vi "Rotation3d_GetXYZ.vi"(11 "in Rotation3d":T1={"Q_quaternion"={"R"=1.0, "V"=[0.0, 0.0, 0.0]}}) -> (1 "Z":dbl, 2 "Y":dbl, 3 "X":dbl)   [LabVIEW 2019, in "Trajectory_Library.lvlib"]
doc: "Returns the counterclockwise rotation angle around the X axis (roll) in radians and the counterclockwise rotation angle around the Y axis (pitch) in radians and the counterclockwise rotation angle around the Z axis (yaw) in radians.\n\nParameters:\n - in ROTATION3D - This ROTATION3D data structure\n\nReturns:\n - X -- The counterclockwise rotation angle around the X axis (roll) in radians.\n - Y -- The counterclockwise rotation angle around the Y axis (pitch) in radians.\n - Z -- The counterclockwise rotation angle around the Z axis (yaw) in radians."
uses:
  Trajectory_Library.lvlib
  TypeDef/ROTATION3D.ctl
  TypeDef/QUATERNION.ctl
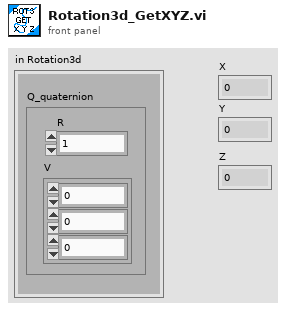
[diagram p1: front panel]
types:
  T1 = typedef "Trajectory_Library.lvlib/ROTATION3D.ctl" = cluster{"Q_quaternion":T2}
  T2 = typedef "Trajectory_Library.lvlib/QUATERNION.ctl" = cluster{"R":dbl, "V":dbl[]}
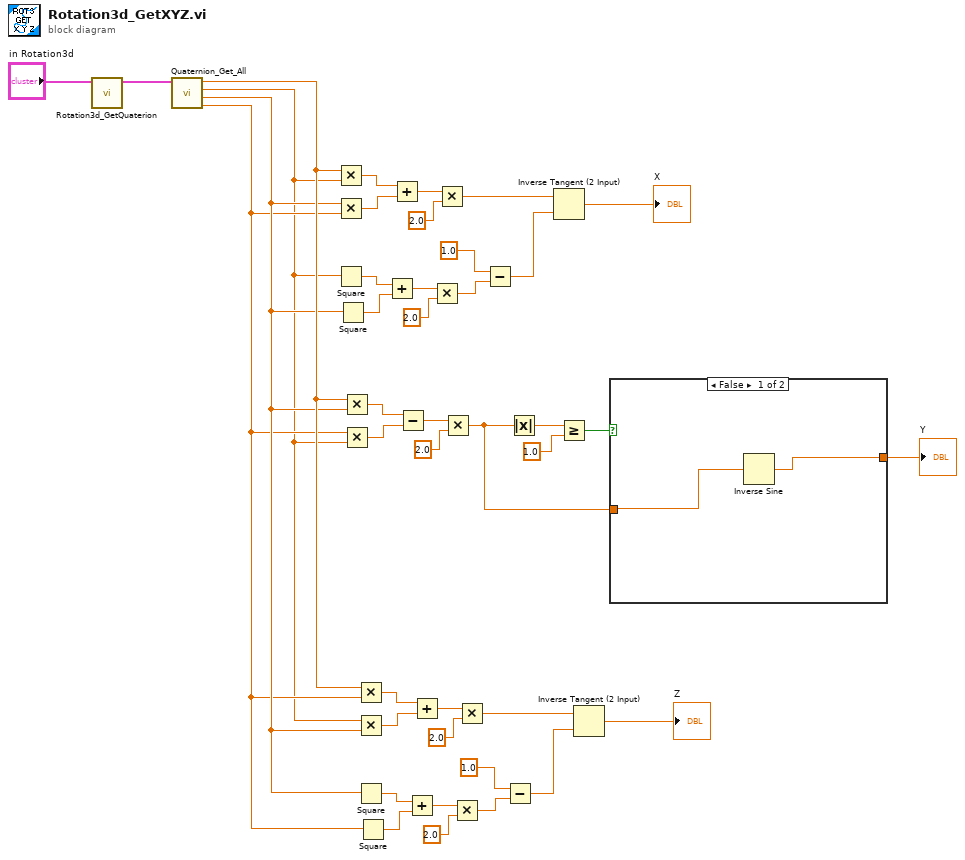
[diagram p0: block diagram]
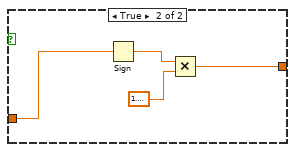
[diagram p2: hidden frame]
diagram:
  n1 = call "Rotation3d_GetQuaterion.vi"("in Rotation3d"="in Rotation3d") -> ("out Quaterion"=w40:T2)  [unwired: 10 in]
  n2 = call "Quaternion_Get_All.vi"("Quaternion"=w40) -> ("Z"=w7:dbl, "Y"=w8:dbl, "X"=w6:dbl, "W"=w9:dbl)  [unwired: 7 in]
  n3 = Multiply(x=w9, y=w6) -> (x*y=w39:dbl)
  n4 = Multiply(x=w8, y=w7) -> (x*y=w38:dbl)
  n5 = Square(x=w6) -> (x^2=w32:dbl)
  n6 = Square(x=w8) -> (x^2=w31:dbl)
  n7 = Multiply(x=w9, y=w8) -> (x*y=w13:dbl)
  n8 = Multiply(x=w7, y=w6) -> (x*y=w12:dbl)
  n9 = Multiply(x=w9, y=w7) -> (x*y=w26:dbl)
  n10 = Multiply(x=w6, y=w8) -> (x*y=w25:dbl)
  n11 = Square(x=w8) -> (x^2=w19:dbl)
  n12 = Square(x=w7) -> (x^2=w18:dbl)
  n13 = Add(x=w32, y=w31) -> (x+y=w34:dbl)
  n14 = Add(x=w39, y=w38) -> (x+y=w37:dbl)
  n15 = Subtract(x=w13, y=w12) -> (x-y=w11:dbl)
  n16 = Add(x=w19, y=w18) -> (x+y=w21:dbl)
  n17 = Add(x=w26, y=w25) -> (x+y=w24:dbl)
  n18 = Multiply(x=w34, y=2.0) -> (x*y=w29:dbl)
  n19 = Multiply(x=w37, y=2.0) -> (x*y=w35:dbl)
  n20 = Multiply(x=w11, y=2.0) -> (x*y=w2:dbl)
  n21 = Multiply(x=w21, y=2.0) -> (x*y=w16:dbl)
  n22 = Multiply(x=w24, y=2.0) -> (x*y=w22:dbl)
  n23 = Subtract(x=1.0, y=w29) -> (x-y=w28:dbl)
  n24 = Subtract(x=1.0, y=w16) -> (x-y=w15:dbl)
  n25 = Absolute Value(x=w2) -> (abs(x)=w5:dbl)
  n26 = Inverse Tangent (2 Input)(1:w28, 2:w35) -> (0:→"X":dbl)
  n27 = Greater Or Equal?(x=w5, y=1.0) -> (x >= y?=w3:bool)
  n28 = Inverse Tangent (2 Input)(1:w15, 2:w22) -> (0:→"Z":dbl)
  n29 = case shown="False" w3 {
    tunnel: w2 -> [w43 w45]
    tunnel: [w42 w44] -> w1
    frame False {
      n30 = Inverse Sine(1:w43) -> (0:w42:dbl)
    }
    frame True {
      n31 = Sign(1:w45) -> (0:w46:dbl)
      n32 = Multiply(x=w46, y=1.5707963267948966) -> (x*y=w44:dbl)
    }
  }
  "Y" <- w1
